vi "PH_IEEE1394Camera.evt call SetBitDepth.vi"(0 "i ref in":refnum<vi>, 2 "Instance":string, 3 "Bit Depth":u32(ring), 5 "error in (no error)":errorcluster) -> (14 "i ref out":refnum<vi>, 19 "error out":errorcluster)   [LabVIEW 2014, in "PH_IEEE1394Camera.lvlib"]
doc: "This VI sends a simple call for SetCamMode."
uses:
  PH_IEEE1394Camera.lvlib
  CSCore/CSSystem/CoreLib/CoreLib.int 2 byte array.vi
  CSCore/CSSystem/CoreLib/CoreLib.lvlib
  CSCore/BaseProcess/BaseProcess.lvlib
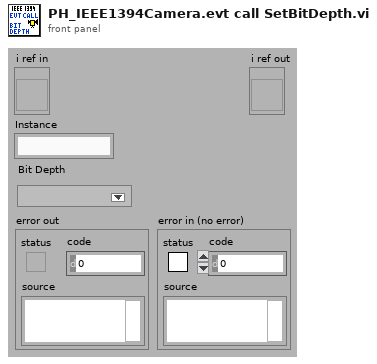
[diagram p1: front panel]
types:
  T1 = typedef "CoreDefs.rawDataType.ctl" = i8[]
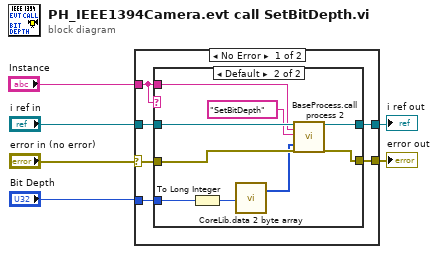
[diagram p0: block diagram]
diagram:
  n1 = case shown="No Error" "error in (no error)" {
    selector: "error in (no error)" -> [w9 w24]
    tunnel: [w12 w25] -> w4
    tunnel: [w11 w24] -> w3
    tunnel: "i ref in" -> [w10 w25]
    tunnel: "Instance" -> [w8 _]
    tunnel: "Bit Depth" -> [w7 _]
    frame No Error {
      n2 = case shown="Default" w8 {
        tunnel: [w14 w23] -> w12
        tunnel: [w13 w22] -> w11
        tunnel: w10 -> [w14 w21]
        tunnel: w8 -> [_ w20]
        tunnel: w9 -> [w13 w18]
        tunnel: w7 -> [_ w16]
        frame "N/A" {
        }
        frame Default {
          n3 = To Long Integer(number=w16) -> (32bit integer=w15:i32)
          n4 = call-poly "CoreLib.data 2 byte array.vi"("i32"=w15) -> ("byteArray out"=w17:T1)  [unwired: 18 in]
          n5 = call "BaseProcess.call process 2.vi"("i ref in"=w21, "Object"=w20, "Selector"="SetBitDepth", "Data"=w17, "error in (no error)"=w18) -> ("i ref out"=w23:refnum<vi>, "error out"=w22:errorcluster)  [unwired: 13 in]
        }
      }
    }
    frame Error {
    }
  }
  "error out" <- w3
  "i ref out" <- w4
